vi "Set Framed Test Node Path.vi"(8 "error in (no error)":errorcluster, 10 "Framed Test Node Path":path, 11 "Edit Test Node Model in":refnum<class "Edit Test Node Model.lvclass">) -> (0 "error out":errorcluster, 3 "Edit Test Node Model out":refnum<class "Edit Test Node Model.lvclass">)   [LabVIEW 2013, in "Edit Test Node Model.lvlib" / "Edit Test Node Model.lvclass"]
uses:
  Edit Test Node Model.lvclass
  Edit Test Node Model.lvclass/Edit Test Node Model.ctl
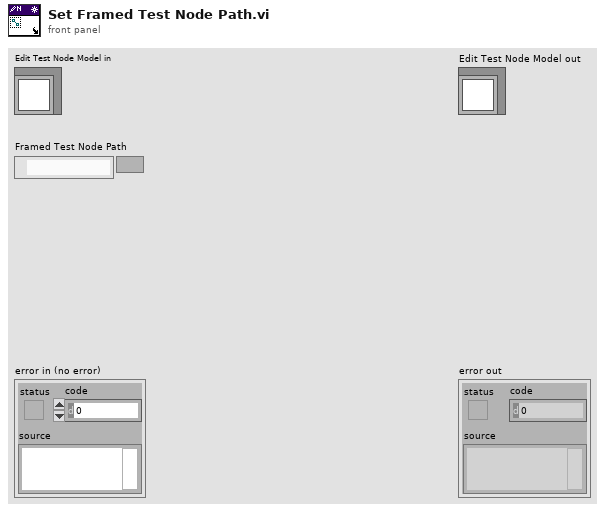
[diagram p1: front panel]
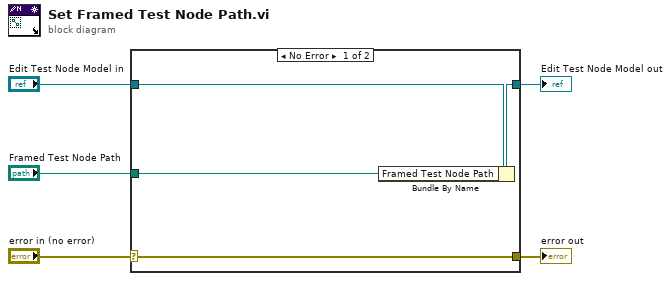
[diagram p0: block diagram]
diagram:
  n1 = case shown="No Error" "error in (no error)" {
    selector: "error in (no error)" -> [w9 w10]
    tunnel: [w9 w10] -> w4
    tunnel: [w7 w11] -> w2
    tunnel: "Edit Test Node Model in" -> [w8 w11]
    tunnel: "Framed Test Node Path" -> [w6 _]
    frame No Error {
      n2 = Bundle By Name(cluster=w8, "Framed Test Node Path"=w6) -> (w7:refnum<class "Edit Test Node Model.lvclass">)
    }
    frame Error {
    }
  }
  "error out" <- w4
  "Edit Test Node Model out" <- w2
